vi "Check_Nested_Loops.vi"(0 "Input Sequence":cluster{string, string[], dbl[], dbl}[](array[cluster])) -> (1 "Syntax Error":bool, 2 "Error Index":i32)   [LabVIEW 2011]
doc: "This VI checks the sequence to ensure that all loops and discrete API commands are properly nested."
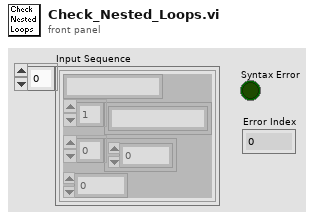
[diagram p1: front panel]
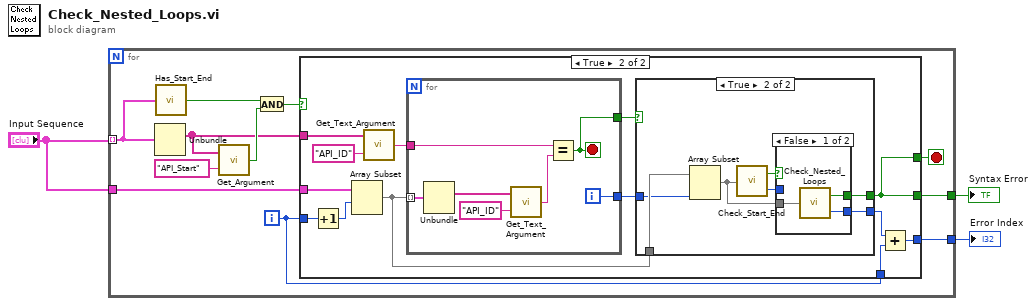
[diagram p0: block diagram]
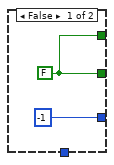
[diagram p2: hidden frame]
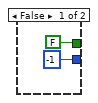
[diagram p3: hidden frame]
diagram:
  n1 = for {
    tunnel: "Input Sequence" -> [w12] mode=indexing
    tunnel: "Input Sequence" -> [w8]
    tunnel: [w6] -> w2
    tunnel: [w4] -> w1
    i -> [w5]
    stop <- w7 stop-if-true
    n2 = Unbundle(w12) -> (w9:string[])  [unwired: 3 out]
    n3 = call "Has_Start_End.vi"("Command"=w12) -> ("Has Start and End"=w11:bool)
    n4 = call "Get_Argument.vi"("Argument"="API_Start", "Argument List"=w9) -> ("Enabled"=w13:bool)
    n5 = And(x=w11, y=w13) -> (x .and. y?=w10:bool)
    n6 = case shown="True" w10 {
      tunnel: w8 -> [_ w29]
      tunnel: w5 -> [_ w27]
      tunnel: w9 -> [_ w26]
      tunnel: [w15 w20] -> w7
      tunnel: [w15 w20] -> w6
      tunnel: [-1 ("Error Index") w19] -> w4
      tunnel: w5 -> [_ w17]
      frame False {
        w15 = FALSE ("Syntax Error")
      }
      frame True {
        n7 = Increment(x=w27) -> (x+1=w28:i32)
        n8 = Array Subset(array=w29, index=w28) -> (w21:cluster{string, string[], dbl[], dbl}[])  [unwired: 1 in]
        n9 = call "Get_Text_Argument.vi"("Argument"="API_ID", "Argument List"=w26) -> ("Text"=w24:string)
        n10 = for {
          tunnel: w21 -> [w49] mode=indexing
          tunnel: w24 -> [w50]
          tunnel: [w45] -> w23
          tunnel: [w44] -> w22
          i -> [w44]
          stop <- w45 stop-if-true
          n11 = Unbundle(w49) -> (w47:string[])  [unwired: 3 out]
          n12 = call "Get_Text_Argument.vi"("Argument"="API_ID", "Argument List"=w47) -> ("Text"=w46:string)
          n13 = Equal?(x=w50, y=w46) -> (x = y?=w45:bool)
        }
        n14 = case shown="True" w23 {
          tunnel: w22 -> [_ w32]
          tunnel: w21 -> [_ w34]
          tunnel: [-1 ("Error Index") w37] -> w18
          tunnel: [FALSE ("Syntax Error") w35] -> w20
          frame False {
          }
          frame True {
            n15 = Array Subset(array=w34, length=w32) -> (w33:cluster{string, string[], dbl[], dbl}[])  [unwired: 1 in]
            n16 = call "Check_Start_End.vi"("Input Sequence"=w33) -> ("Syntax Error"=w38:bool, "Error Index"=w36:i32)
            n17 = case shown="False" w38 {
              selector: w38 -> [_ w42]
              tunnel: w33 -> [w41 _]
              tunnel: [w40 w42] -> w35
              tunnel: [w39 w43] -> w37
              tunnel: w36 -> [_ w43]
              frame False {
                n18 = call "Check_Nested_Loops.vi"("Input Sequence"=w41) -> ("Syntax Error"=w40:bool, "Error Index"=w39:i32)
              }
              frame True {
              }
            }
          }
        }
        n19 = Add(x=w18, y=w17) -> (x+y=w19:i32)
      }
    }
  }
  "Error Index" <- w1
  "Syntax Error" <- w2
